vi "ADS Errors.vi"(8 "error in (no error)":errorcluster, 11 "ADS Error":T1 items=["NoError"=0, "InternalError"=1, "NoRTime"=2, "LockedMemoryError"=3, "MailBoxError"=4, "WrongHMsg"=5, "TargetPortNotFound"=6, "TargetMachineNotFound"=7, "UnknownCommandID"=8, "BadTaskID"=9, "NoIO"=10, "UnknownAmsCommand"=11, "Win32Error"=12, "PortNotConnected"=13, "InvalidAmsLength"=14, "InvalidAmsNetID"=15, "AmsSyncAmsError"=22, "AmsSyncNoIndexMap"=23, "InvalidAmsPort"=24, "NoMemory"=25, "TCPSendError"=26, "HostUnreachable"=27, "NoLockedMemory"=1280, "MailboxFull"=1282, "DeviceError"=1792, "DeviceServiceNotSupported"=1793, "DeviceInvalidGroup"=1794, "DeviceInvalidOffset"=1795, "DeviceInvalidAccess"=1796, "DeviceInvalidSize"=1797, "DeviceInvalidData"=1798, "DeviceNotReady"=1799, "DeviceBusy"=1800, "DeviceInvalidContext"=1801, "DeviceNoMemory"=1802, "DeviceInvalidParam"=1803, "DeviceNotFound"=1804, "DeviceSyntaxError"=1805, "DeviceIncompatible"=1806, "DeviceExists"=1807, "DeviceSymbolNotFound"=1808, "DeviceSymbolVersionInvalid"=1809, "DeviceInvalidState"=1810, "DeviceTransModeNotSupported"=1811, "DeviceNotifyHandleInvalid"=1812, "DeviceClientUnknown"=1813, "DeviceNoMoreHandles"=1814, "DeviceInvalidWatchsize"=1815, "DeviceNotInitialized"=1816, "DeviceTimeOut"=1817, "DeviceNoInterface"=1818, "DeviceInvalidInterface"=1819, "DeviceInvalidCLSID"=1820, "DeviceInvalidObjectID"=1821, "ClientError"=1856, "ClientInvalidParameter"=1857, "ClientListEmpty"=1858, "ClientVariableInUse"=1859, "ClientDuplicateInvokeID"=1860, "ClientSyncTimeOut"=1861, "ClientW32OR"=1862, "ClientTimeoutInvalid"=1863, "ClientPortNotOpen"=1864, "ClientNoAmsAddr"=1865, "ClientSyncInternal"=1872, "ClientAddHash"=1873, "ClientRemoveHash"=1874, "ClientNoMoreSymbols"=1875, "ClientSyncResInvalid"=1876, "ClientSyncPortLocked"=1877, "ClientQueueFull"=1878]) -> (0 "error out":errorcluster)   [LabVIEW 2017, in "TwinCAT ADS.lvlib" / "PLC.lvlib"]
uses:
  High Level/PLC/PLC.lvlib
  TypeDefs/ADS Error.ctl
  <vilib>/ErrorRing/Error Ring.xnode
  TwinCAT ADS.lvlib
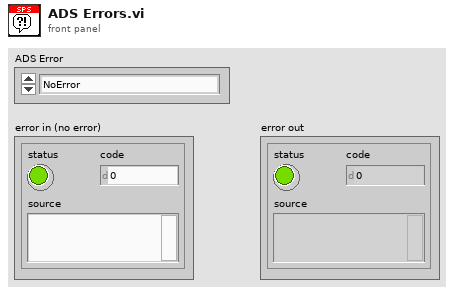
[diagram p1: front panel]
types:
  T1 = typedef "TwinCAT ADS.lvlib/ADS Error.ctl" = i32
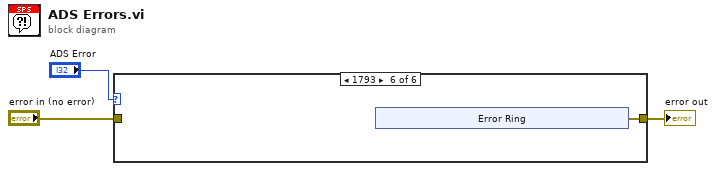
[diagram p0: block diagram]
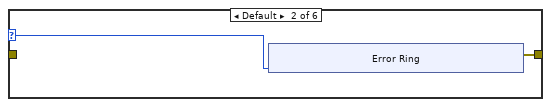
[diagram p3: hidden frame]
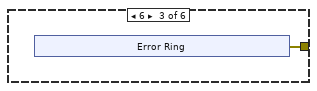
[diagram p4: hidden frame]
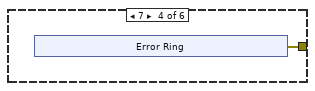
[diagram p5: hidden frame]
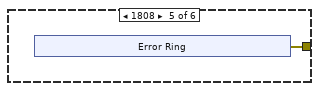
[diagram p6: hidden frame]
diagram:
  n1 = case shown="1793" "ADS Error" {
    selector: "ADS Error" -> [_ w5 _ _ _ _]
    tunnel: "error in (no error)" -> [w4 _ _ _ _ _]
    tunnel: [w4 w6 w12 w14 w16 w18] -> w3
    frame 0 {
    }
    frame Default {
      n2 = xnode "Error Ring"("parameter 0"=w5) -> ("error out"=w6:errorcluster)
    }
    frame 6 {
      n3 = xnode "Error Ring"() -> ("error out"=w12:errorcluster)
    }
    frame 7 {
      n4 = xnode "Error Ring"() -> ("error out"=w14:errorcluster)
    }
    frame 1808 {
      n5 = xnode "Error Ring"() -> ("error out"=w16:errorcluster)
    }
    frame 1793 {
      n6 = xnode "Error Ring"() -> ("error out"=w18:errorcluster)
    }
  }
  "error out" <- w3
